vi "Deadband calcualations.vi"(7 "Turn Only":bool, 8 "From shift time":u32, 9 "Deadbands":T1, 10 "Procces Variables":cluster{"Angle":dbl, "Encoder Distance":dbl}, 11 "Setpoints":T2) -> (0 "to shift time":u32, 2 "In Range":bool, 3 "In Range in time":bool)   [LabVIEW 2013]
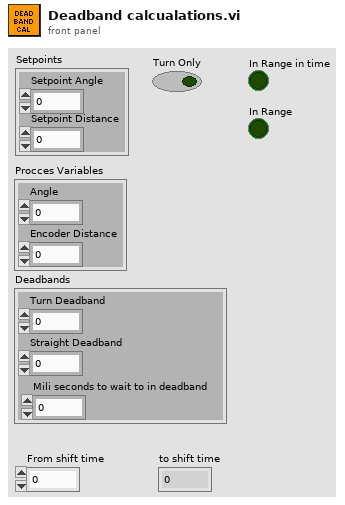
[diagram p1: front panel]
types:
  T1 = cluster{"Turn Deadband":dbl, "Straight Deadband":dbl, "Mili seconds to wait to in deadband":u32}
  T2 = cluster{"Setpoint Angle":dbl, "Setpoint Distance":dbl}
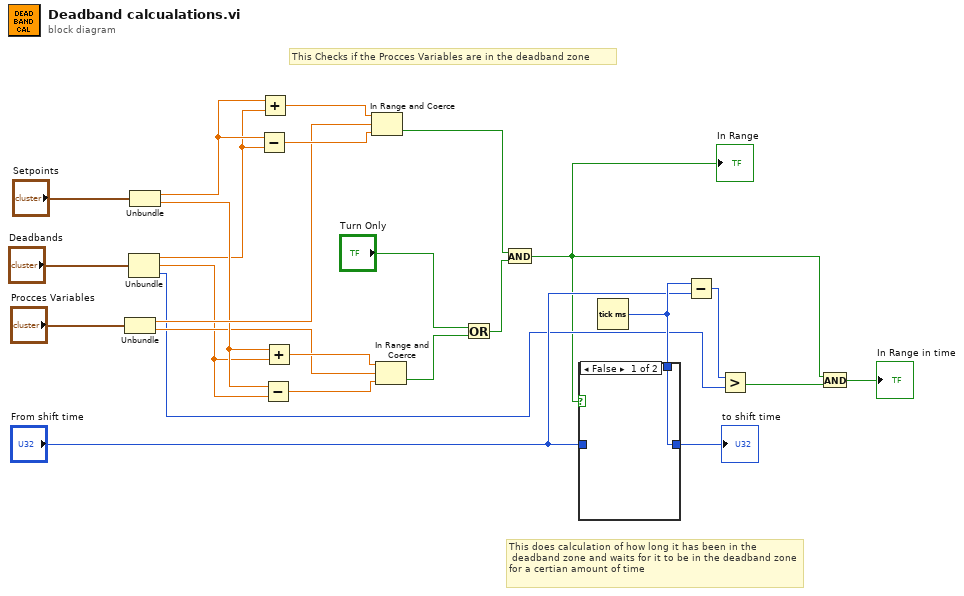
[diagram p0: block diagram]
diagram:
  # "This does calculation of how long it has been in the\n deadband zone and waits for it to be in the deadband zone for a certian amount of time"
  # "This Checks if the Procces Variables are in the deadband zone"
  n1 = Unbundle("Procces Variables") -> ("Angle"=w20:dbl, "Encoder Distance"=w16:dbl)
  n2 = Unbundle("Deadbands") -> ("Turn Deadband"=w10:dbl, "Straight Deadband"=w9:dbl, "Mili seconds to wait to in deadband"=w4:u32)
  n3 = Unbundle("Setpoints") -> ("Setpoint Angle"=w25:dbl, "Setpoint Distance"=w17:dbl)
  n4 = Subtract(x=w25, y=w10) -> (x-y=w23:dbl)
  n5 = Add(x=w25, y=w10) -> (x+y=w24:dbl)
  n6 = Subtract(x=w17, y=w9) -> (x-y=w18:dbl)
  n7 = Add(x=w17, y=w9) -> (x+y=w19:dbl)
  n8 = In Range and Coerce(upper limit=w24, x=w20, lower limit=w23) -> (In Range?=w12:bool)  [unwired: 1 out]
  n9 = In Range and Coerce(upper limit=w19, x=w16, lower limit=w18) -> (In Range?=w14:bool)  [unwired: 1 out]
  n10 = Or(x="Turn Only", y=w14) -> (x .or. y?=w13:bool)
  n11 = And(x=w12, y=w13) -> (x .and. y?=w1:bool)
  "In Range" <- w1
  n12 = Tick Count (ms)() -> (millisecond timer value=w8:u32)
  n13 = case shown="False" w1 {
    tunnel: "From shift time" -> [_ w27]
    tunnel: w8 -> [w26 _]
    tunnel: [w26 w27] -> w6
    frame False {
    }
    frame True {
    }
  }
  "to shift time" <- w6
  n14 = Subtract(x=w8, y="From shift time") -> (x-y=w5:u32)
  n15 = Greater?(x=w5, y=w4) -> (0:w2:bool)
  n16 = And(x=w1, y=w2) -> (x .and. y?=→"In Range in time":bool)
